vi "Start High-Speed Data Communication.vi"(0 "Device ID (0)":i32, 1 "Max Buffer Size":u32, 5 "Comm Interface":T1, 7 "Ethernet Config":T2={"IP Address"=[192, 168, 0, 1], "Port No"=24692}, 9 "Start Req":T3={"High-Speed Comm Start Pos"=0, "Read Profile Cnt"=0, "High-Speed Receive Ratio"=16} {"High-Speed Receive Ratio" items=["LOWEST"=0, "LOW"=16, "MIDDLE"=17, "HIGH"=18, "HIGHEST"=32]; "High-Speed Comm Start Pos" items=["SEND COMPLETE POS", "OLDEST", "NEXT"]}, 11 "error in (no error)":errorcluster) -> (4 "Device ID out":i32, 15 "error out":errorcluster)   [LabVIEW 2014, in "Keyence LJ-V7000.lvlib"]
doc: "High-speed communication with the controller is established to start.\n\n<B>Note</B>: \nIf one packet of profiles of high-speed communication are not received for 30 seconds during high-speed data communication, high-speed data communication will be terminated due to time-out."
uses:
  Keyence LJ-V7000.lvlib
  Clusters/High-Speed Comm Start Req.ctl
  constant/High-Speed Comm Start Pos.ctl
  constant/High-Speed Receive Ratio.ctl
  Clusters/Ethernet Config.ctl
  constant/Comm Interface.ctl
  constant/Driver VI No.ctl
panel:
  # "(c) 2012 KEYENCE CORPORATION.  ALL RIGHTS RESERVED."
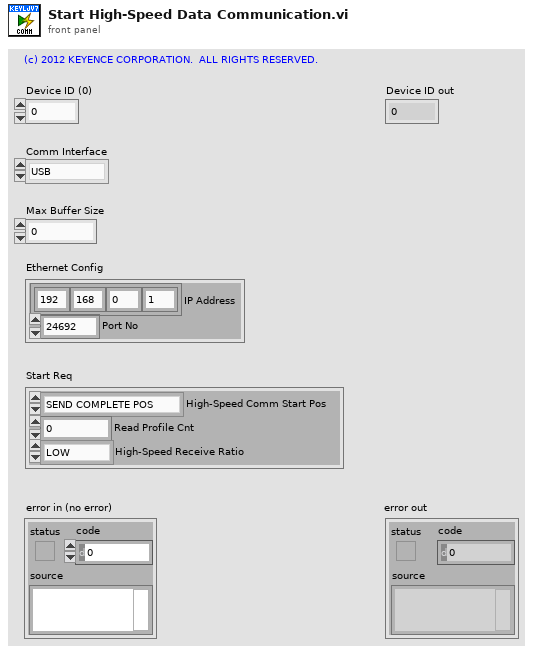
[diagram p1: front panel]
types:
  T1 = typedef "Keyence LJ-V7000.lvlib/Comm Interface.ctl" = enum8{"USB", "ETHERNET"}
  T2 = typedef "Keyence LJ-V7000.lvlib/Ethernet Config.ctl" = cluster{"IP Address":u8[], "Port No":u16}
  T3 = typedef "Keyence LJ-V7000.lvlib/High-Speed Comm Start Req.ctl" = cluster{"High-Speed Comm Start Pos":T4, "Read Profile Cnt":u32, "High-Speed Receive Ratio":T5}
  T4 = typedef "Keyence LJ-V7000.lvlib/High-Speed Comm Start Pos.ctl" = u8
  T5 = typedef "Keyence LJ-V7000.lvlib/High-Speed Receive Ratio.ctl" = u8
  T6 = typedef "Keyence LJ-V7000.lvlib/Driver VI No.ctl" = enum16{"Initialize", "Close", "Reboot Controller", "Return to Factory State", "Get System Error", "Clear System Error", "Trigger", "Start Batch Measurements", "Stop Batch Measurements", "Auto Zero", "Timing", "Reset", "Clear Memory", "Set Setting", "Get Setting", "Initialize Setting", "Reflect Setting", "Update Write Settings Area", "Check Status of Saving to Save Area", "Set Time", "Get Time", "Change Program", "Read Active Program Number", "Read Measurement Data", "Read Profiles(for High-Speed Mode)", "Read Batch Profiles(for High-Speed Mode)", "Read Profiles(for Advanced Mode)", "Read Batch Profiles(for Advanced Mode)", "Start Storage", "Stop Storage", "Read Storage Status", "Read Data Storage Data", "Read Profile Storage Data", "Read Batch Profile Storage Data", "Start High-Speed Data Communication", "Stop High-Speed Data Communication", "Read Profiles(for High-Speed Communication)"}
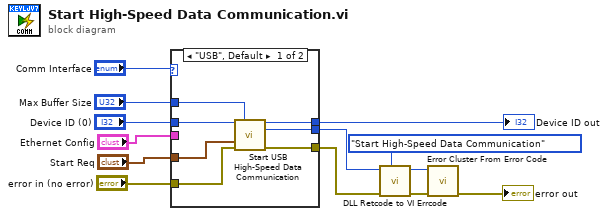
[diagram p0: block diagram]
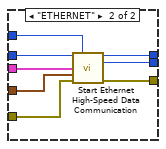
[diagram p2: hidden frame]
diagram:
  n1 = case shown="\"USB\", Default" "Comm Interface" {
    tunnel: "Max Buffer Size" -> [w20 w28]
    tunnel: "Device ID (0)" -> [w19 w27]
    tunnel: "Start Req" -> [w18 w26]
    tunnel: "error in (no error)" -> [w17 w25]
    tunnel: "Ethernet Config" -> [_ w24]
    tunnel: [w16 w23] -> w7
    tunnel: [w15 w22] -> w4
    tunnel: [w14 w21] -> w3
    frame "USB", Default {
      n2 = call "Start USB High-Speed Data Communication.vi"("Device ID"=w19, "Max Buffer Size"=w20, "Start Req"=w18, "error in (no error)"=w17) -> ("Device ID out"=w16:i32, "Return Code"=w15:i32, "error out"=w14:errorcluster)  [unwired: 9 in]
    }
    frame "ETHERNET" {
      n3 = call "Start Ethernet High-Speed Data Communication.vi"("Device ID"=w27, "Max Buffer Size"=w28, "Ethernet Config"=w24, "Start Req"=w26, "error in (no error)"=w25) -> ("Device ID out"=w23:i32, "Return Code"=w22:i32, "error out"=w21:errorcluster)  [unwired: 8 in]
    }
  }
  "Device ID out" <- w7
  n4 = call "DLL Retcode to VI Errcode.vi"("Driver VI No"=Driver_VI_No."Start High-Speed Data Communication", "error in (no error)"=w3, "DLL Return Code"=w4) -> ("error out"=w6:errorcluster, "VI Error Code"=w5:i32)  [unwired: 7 in]
  n5 = call <vilib>:"Error Cluster From Error Code.vi"("error in (no error)"=w6, "error code (0)"=w5) -> ("error out"=→"error out":errorcluster)  [unwired: 7 in]
